vi "ContMotionFixPRF_ESP.vi"(5 "Motion Settings":T1={"No Motion?"=FALSE, "Motion System"=enum."NI 735x", "Motion Bd ID"=1, "Motion Profile"="SMAC1", "# Axis"=1, "Reverse Z axis?"=TRUE, "SMAC Axis"=0, "scan pair"=enum."y-(x) scan", "RT fps"=6.0, "Steps per mm"=[1000, 1000, 1000, 1000], "Motor Parameters"={"velocity ct/s"=[10000.0, 10000.0, 10000.0, 50000.0], "accel ct/s^2"=[50000.0, 50000.0, 50000.0, 200000.0]}, "One Way Scan"=FALSE, "Reverse One Way Scan"=FALSE, "Global Position (mm)"=[], "Plane"=0, "Distance between\nscan lines (um)"=0.0, "Distance between\nscan planes (um)"=0.0, "number of scan planes"=1, "Total steps in line"=0, "Xtra plane\ndistance  (um)"=100, "Xtra planes "=1, "Add Axis"=FALSE, "overshoot cts"=200, "BKPT Shift"=0, "Scan Start Time (ms)"=0, "ESP VISA"="GPIB::1::INSTR", "3rd Axis"=1, "GL Ref Out"=refnum, "Galil Address"=""} {"3rd Axis" items=["x", "y", "z", "w"]; "Xtra planes" min=1; "Xtra plane\ndistance  (um)" min=0; "Distance between\nscan planes (um)" format="%.2f"; "Distance between\nscan lines (um)" format="%.2f"; "SMAC Axis" items=["None"=0, "Axis 1"=1, "Axis 2"=2, "Axis 3"=3, "Axis 4"=4, "Axis 5"=5, "Axis 6"=6, "Axis 7"=7, "Axis 8"=8, "Vector Space 1"=17, "Vector Space 2"=18, "Vector Space 3"=19, "Vector Space 4"=20]; "Motion Bd ID" min=1 max=32 step=1}, 6 "Offset":i32, 7 "Reverse ?":bool, 8 "error in (no error)":errorcluster, 9 "Axis":i32=1 min=1 max=4, 11 "VISA resource name":refnum<visa-resource-name>) -> (0 "error out":errorcluster, 3 "VISA resource name out":refnum<visa-resource-name>)   [LabVIEW 2022 SP3]
uses:
  NI_controller/-NI_MotionRoutines/MotionParameters.ctl
  NI_controller/-NI_MotionRoutines/MotionSys.ctl
  -MotionRoutines/ScanAxis.ctl
  -MotionRoutines/3rdAxis.ctl
  Pulsers/PulserGlobals.vi
  <instrlib>/Newport ESP301/Newport ESP301.lvlib
panel:
  # "1-D and 2-D B scan settings"
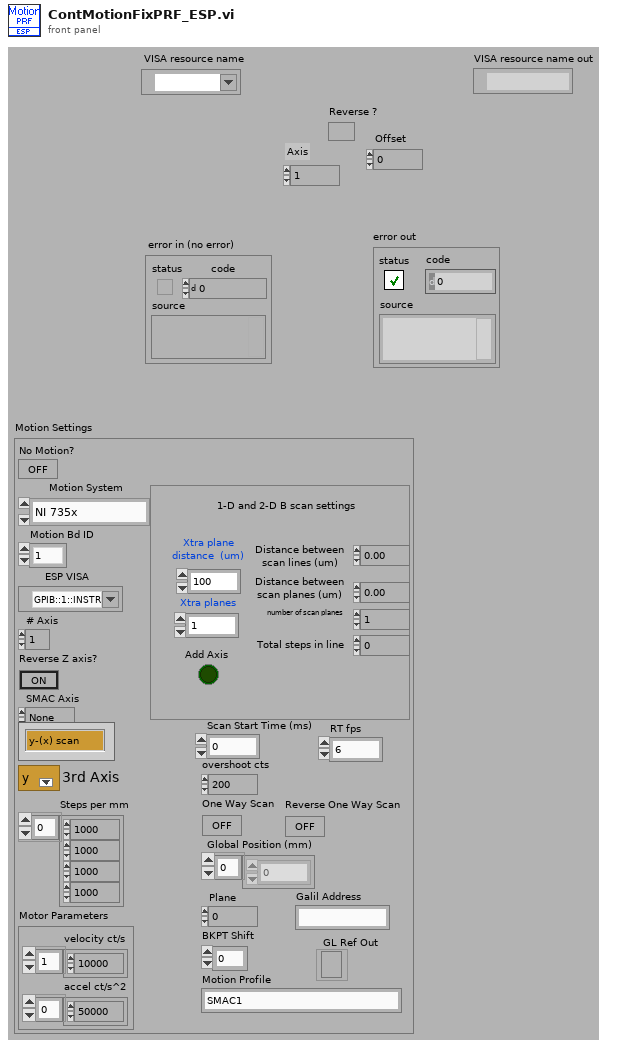
[diagram p1: front panel]
types:
  T1 = typedef "MotionParameters.ctl" = cluster{"No Motion?":bool, "Motion System":T2, "Motion Bd ID":u8, "Motion Profile":string, "# Axis":i8, "Reverse Z axis?":bool, "SMAC Axis":u16, "scan pair":T3, "RT fps":sgl, "Steps per mm":i32[], "Motor Parameters":cluster{"velocity ct/s":dbl[], "accel ct/s^2":dbl[]}, "One Way Scan":bool, "Reverse One Way Scan":bool, "Global Position (mm)":dbl[], "Plane":i32, "Distance between\nscan lines (um)":sgl, "Distance between\nscan planes (um)":sgl, "number of scan planes":i32, "Total steps in line":i32, "Xtra plane\ndistance  (um)":i32, "Xtra planes ":i32, "Add Axis":bool, "overshoot cts":i32, "BKPT Shift":i32, "Scan Start Time (ms)":u32, "ESP VISA":refnum<visa-resource-name>, "3rd Axis":T4, "GL Ref Out":refnum<k7>, "Galil Address":string}
  T2 = typedef "MotionSys.ctl" = enum16{"MM3000", "NI 735x", "Newport ESP", "No Motion Card", "Galil"}
  T3 = typedef "ScanAxis.ctl" = enum16{"y-(x) scan", "x-(y) scan", "z-(x) scan", "z-(y) scan", "y-(z) scan", "x-(z) scan", "w-(x) scan", "w-(y) scan", "w-(z) scan", "x-(w) scan", "y-(w) scan", "z-(w) scan"}
  T4 = typedef "3rdAxis.ctl" = u16
  T5 = cluster{"Port A bit-0 at logic level":bool, "Port A bit-1 at logic level":bool, "Port A bit-2 at logic level ":bool, "Port A bit-3 at logic level":bool, "Port A bit-4 at logic level":bool, "Port A bit-5 at logic level ":bool, "Port A bit-6 at logic level ":bool, "Port A bit-7 at logic level ":bool, "Port B bit-0 at logic level":bool, "Port B bit-1 at logic level":bool, "Port B bit-2 at logic level ":bool, "Port B bit-3 at logic level":bool, "Port B bit-4 at logic level":bool, "Port B bit-5 at logic level ":bool, "Port B bit-6 at logic level ":bool, "Port B bit-7 at logic level ":bool}
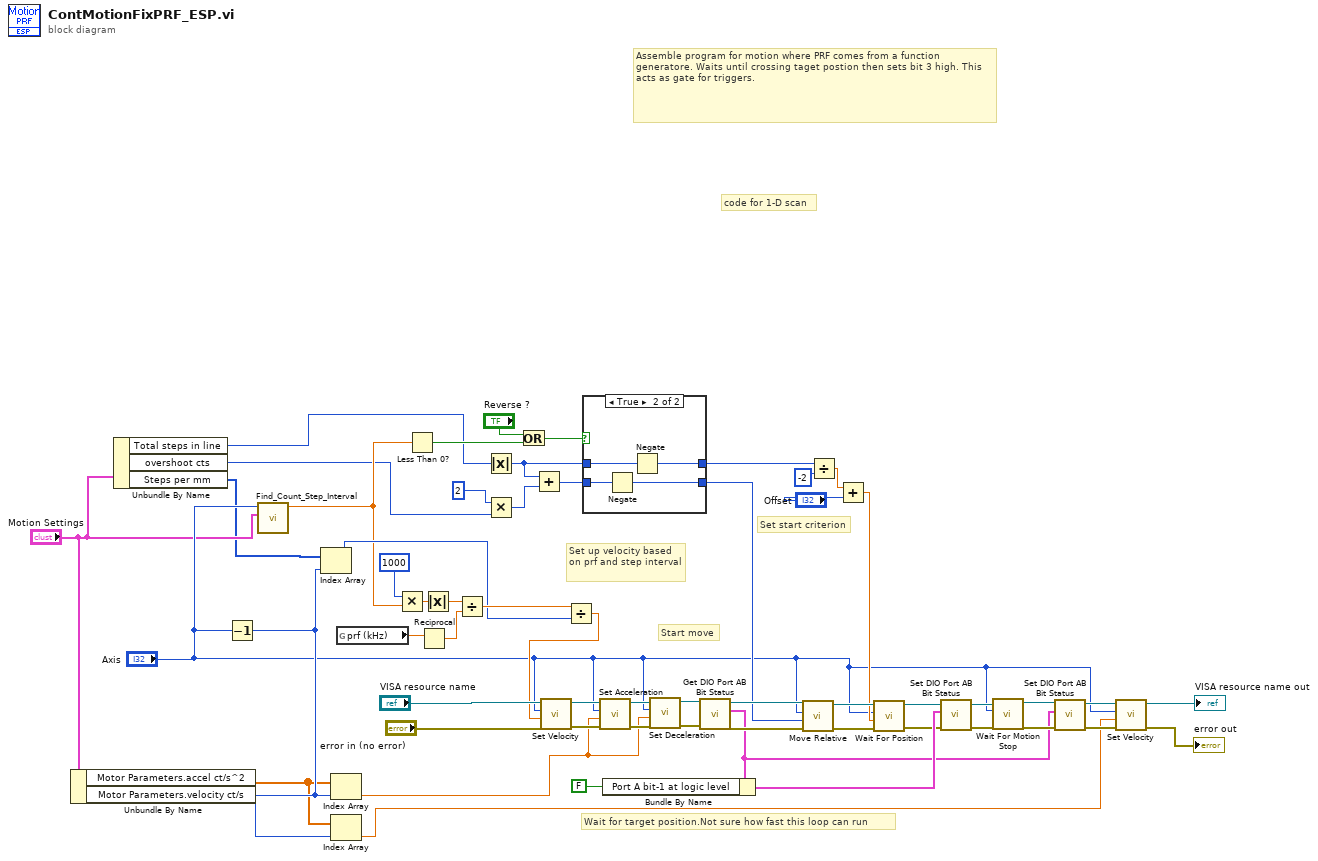
[diagram p0: block diagram]
diagram:
  # "Wait for target position.Not sure how fast this loop can run"
  # "Set start criterion"
  # "Set up velocity based on prf and step interval"
  # "Start move"
  # "code for 1-D scan"
  # "Assemble program for motion where PRF comes from a function generatore. Waits until crossing taget postion then sets bit 3 high. This acts as gate for triggers."
  n1 = Unbundle By Name("Motion Settings") -> ("Motor Parameters.accel ct/s^2"=w9:dbl[])  [unwired: 1 out]
  n2 = Unbundle By Name("Motion Settings") -> ("Total steps in line"=w3:i32, "overshoot cts"=w5:i32, "Steps per mm"=w2:i32[])
  n3 = Decrement(x="Axis") -> (x-1=w10:i32)
  n4 = call "Find_Count_Step_Interval.vi"("Motion Settings In"="Motion Settings", "Axis"="Axis") -> ("BP Interval"=w7:dbl)  [unwired: 8 in, 1 out]
  n5 = Index Array(array=w2, index=w10) -> (element=w12:i32)
  n6 = Index Array(array=w9, index=w10) -> (element=w11:dbl)
  n7 = Index Array(array=w9, index=w10) -> (element=w8:dbl)
  n8 = global read "PulserGlobals.vi" "prf (kHz)"() -> (w1:dbl)
  n9 = Multiply(x=1000, y=w7) -> (x*y=w45:dbl)
  n10 = Less Than 0?(x=w7) -> (x < 0?=w56:bool)
  n11 = Reciprocal(x=w1) -> (1/x=w47:dbl)
  n12 = Absolute Value(x=w45) -> (abs(x)=w52:dbl)
  n13 = Divide(x=w52, y=w47) -> (x/y=w14:dbl)
  n14 = Absolute Value(x=w3) -> (abs(x)=w51:i32)
  n15 = Multiply(x=2, y=w5) -> (x*y=w43:i32)
  n16 = Or(x="Reverse ?", y=w56) -> (x .or. y?=w54:bool)
  n17 = Add(x=w51, y=w43) -> (x+y=w53:i32)
  n18 = Divide(x=w14, y=w12) -> (x/y=w13:dbl)
  n19 = call <instrlib>:"Set Velocity.vi"("error in (no error)"="error in (no error)", "Velocity (units/s)"=w13, "Axis (1)"="Axis", "VISA resource name"="VISA resource name") -> ("error out"=w39:errorcluster, "VISA resource name out"=w40:refnum<visa-resource-name>)  [unwired: 2 in]
  n20 = case shown="True" w54 {
    tunnel: w53 -> [w58 w62]
    tunnel: [w58 w61] -> w27
    tunnel: [w57 w59] -> w48
    tunnel: w51 -> [w57 w60]
    frame False {
    }
    frame True {
      n21 = Negate(x=w62) -> (-x=w61:i32)
      n22 = Negate(x=w60) -> (-x=w59:i32)
    }
  }
  n23 = call <instrlib>:"Set Acceleration.vi"("error in (no error)"=w39, "Acceleration (0 units/s²)"=w11, "Axis (1)"="Axis", "VISA resource name"=w40) -> ("error out"=w42:errorcluster, "VISA resource name out"=w41:refnum<visa-resource-name>)  [unwired: 2 in]
  n24 = call <instrlib>:"Set Deceleration.vi"("error in (no error)"=w42, "Deceleration (0 units/s²)"=w11, "Axis (1)"="Axis", "VISA resource name"=w41) -> ("error out"=w38:errorcluster, "VISA resource name out"=w37:refnum<visa-resource-name>)  [unwired: 2 in]
  n25 = call <instrlib>:"Get DIO Port AB Bit Status.vi"("error in (no error)"=w38, "VISA resource name"=w37) -> ("error out"=w35:errorcluster, "DIO Port A status"=w21:T5, "VISA resource name out"=w36:refnum<visa-resource-name>)  [unwired: 3 in]
  n26 = Bundle By Name(cluster=w21, "Port A bit-1 at logic level"=FALSE ("Port A bit-0 at logic level")) -> (w31:T5)
  n27 = call <instrlib>:"Move Relative.vi"("error in (no error)"=w35, "Position (0 units)"=w27, "Axis (1)"="Axis", "VISA resource name"=w36) -> ("error out"=w30:errorcluster, "VISA resource name out"=w29:refnum<visa-resource-name>)  [unwired: 2 in]
  n28 = Divide(x=w48, y=-2) -> (x/y=w49:dbl)
  n29 = Add(x=w49, y="Offset") -> (x+y=w28:dbl)
  n30 = call <instrlib>:"Wait For Position.vi"("error in (no error)"=w30, "Position (0 units)"=w28, "Axis (1)"="Axis", "VISA resource name"=w29) -> ("error out"=w24:errorcluster, "VISA resource name out"=w25:refnum<visa-resource-name>)  [unwired: 2 in]
  n31 = call <instrlib>:"Set DIO Port AB Bit Status.vi"("error in (no error)"=w24, "DIO Port status"=w31, "VISA resource name"=w25) -> ("error out"=w16:errorcluster, "VISA resource name out"=w17:refnum<visa-resource-name>)  [unwired: 3 in]
  n32 = call <instrlib>:"Wait For Motion Stop.vi"("error in (no error)"=w16, "Axis (0)"="Axis", "VISA resource name"=w17) -> ("error out"=w22:errorcluster, "VISA resource name out"=w23:refnum<visa-resource-name>)  [unwired: 3 in]
  n33 = call <instrlib>:"Set DIO Port AB Bit Status.vi"("error in (no error)"=w22, "DIO Port status"=w21, "VISA resource name"=w23) -> ("error out"=w19:errorcluster, "VISA resource name out"=w20:refnum<visa-resource-name>)  [unwired: 3 in]
  n34 = call <instrlib>:"Set Velocity.vi"("error in (no error)"=w19, "Velocity (units/s)"=w8, "Axis (1)"="Axis", "VISA resource name"=w20) -> ("error out"=→"error out":errorcluster, "VISA resource name out"=→"VISA resource name out":refnum<visa-resource-name>)  [unwired: 2 in]
